vi "FF_SagittalTo3D.vi"(2 "AnkleInGCS":dbl[](array[numeric]), 3 "ForceInXY":dbl[](array[numeric])) -> (1 "ForceInXYZ":dbl[](array[numeric]))   [LabVIEW 2016, in "ForceField.lvclass"]
uses:
  ForceField.lvclass
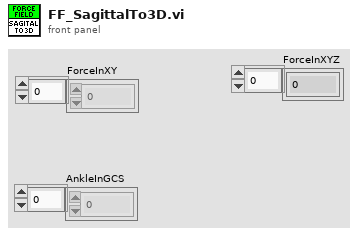
[diagram p1: front panel]
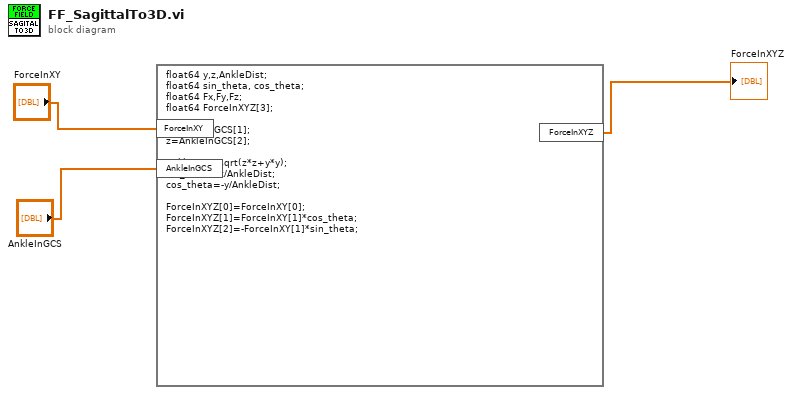
[diagram p0: block diagram]
diagram:
  n1 = formula code="float64 y,z,AnkleDist;\nfloat64 sin_theta, cos_theta;\nfloat64 Fx,Fy,Fz;\nfloat64 ForceInXYZ[3];\n\ny=AnkleInGCS[1];\nz=AnkleInGCS[2];\n\nAnkleDist=sqrt(z*z+y*y);\nsin_theta=z/AnkleDist;\ncos_theta=-y/AnkleDist;\n\nForceInXYZ[0]=ForceInXY[0];\nForceInXYZ[1]=ForceInXY[1]*cos_theta;\nForceInXYZ[2]=-ForceInXY[1]*sin_theta;"("ForceInXY"="ForceInXY", "AnkleInGCS"="AnkleInGCS") -> ("ForceInXYZ"=→"ForceInXYZ":dbl[])
